vi "Reset UI.vi"(8 "error in (no error)":errorcluster, 11 "BuildServer in":refnum<class "BuildServer.lvclass">) -> (0 "error out":errorcluster, 3 "BuildServer out":refnum<class "BuildServer.lvclass">)   [LabVIEW 2017, in "BuildServer.lvlib" / "BuildServer.lvclass"]
uses:
  BuildServer.lvclass
  ProjectOrganization.ctl
  BuildServer.lvclass/BuildServer.ctl
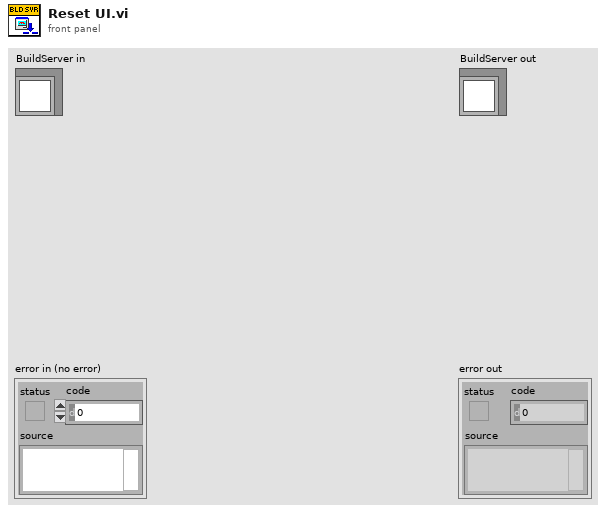
[diagram p1: front panel]
types:
  T1 = typedef "BuildServer.lvlib/BuildServer.lvclass/ProjectOrganization.ctl" = enum16{"Group by Project", "Group by Target", "Group by Type", "Group by Name"}
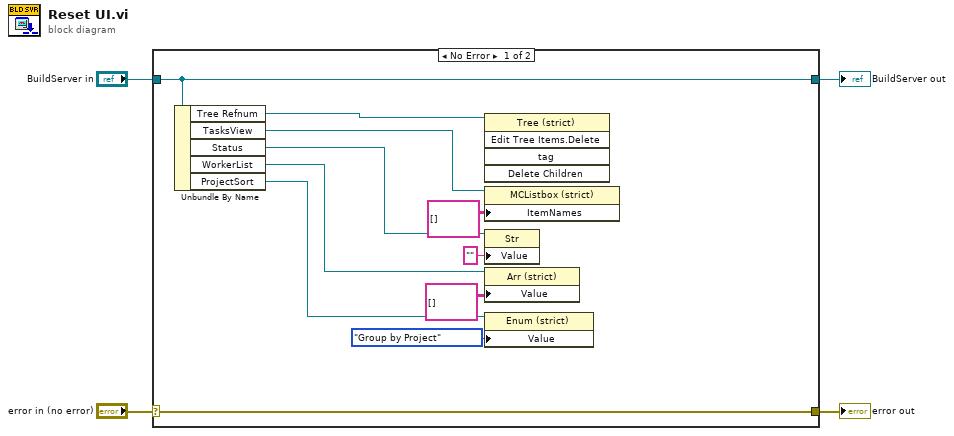
[diagram p0: block diagram]
diagram:
  n1 = case shown="No Error" "error in (no error)" {
    selector: "error in (no error)" -> [w15 w17]
    tunnel: [w15 w17] -> w3
    tunnel: [w5 w16] -> w1
    tunnel: "BuildServer in" -> [w5 w16]
    frame No Error {
      n2 = Unbundle By Name(w5) -> ("Tree Refnum"=w14:refnum<vi>, "TasksView"=w13:refnum<vi>, "Status"=w11:refnum<vi>, "WorkerList"=w9:refnum<vi>, "ProjectSort"=w7:refnum<vi>)
      n3 = invoke class="Tree (strict)" method="Edit Tree Items.Delete"(reference=w14) -> ()  [unwired: 4 in, 5 out]
      n4 = property class="MCListbox (strict)"(reference=w13, "ItemNames"=string[][] [] ("Item Names")) -> ()  [unwired: 1 in, 2 out]
      n5 = property class="Str"(reference=w11, "Value"="") -> ()  [unwired: 1 in, 2 out]
      n6 = property class="Arr (strict)"(reference=w9, "Value"=string[][] []) -> ()  [unwired: 1 in, 2 out]
      n7 = property class="Enum (strict)"(reference=w7, "Value"=ProjectOrganization."Group by Project") -> ()  [unwired: 1 in, 2 out]
    }
    frame Error {
    }
  }
  "error out" <- w3
  "BuildServer out" <- w1
